vi "IPI_Value Test.vi"(8 "Stand":dbl, 9 "下限":dbl, 10 "上限":dbl, 11 "input":dbl format="%#_13g") -> (3 "output value":dbl)   [LabVIEW 2015]
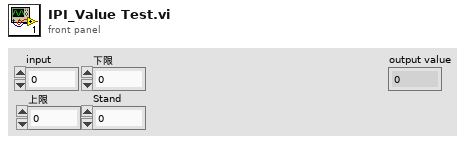
[diagram p1: front panel]
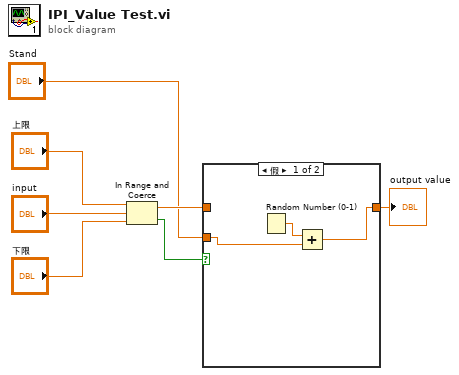
[diagram p0: block diagram]
diagram:
  n1 = In Range and Coerce(upper limit="上限", x="input", lower limit="下限") -> (coerced(x)=w3:dbl, In Range?=w4:bool)
  n2 = case shown="假" w4 {
    tunnel: w3 -> [_ w11]
    tunnel: [w8 w11] -> w2
    tunnel: "Stand" -> [w9 _]
    frame False {
      n3 = Random Number (0-1)() -> (number: 0 to 1=w10:dbl)
      n4 = Add(x=w10, y=w9) -> (x+y=w8:dbl)
    }
    frame True {
    }
  }
  "output value" <- w2
